vi "Configure Rx Parameters.vi"(6 "rx_gains":dbl[](array[numeric]), 7 "rx_freqs":dbl[](array[numeric]), 8 "error in (no error)":errorcluster, 9 "python path":path, 10 "session in":refnum<k38>, 11 "Refnum in":refnum<k35>) -> (0 "error out":errorcluster, 1 "rx_freqs out":dbl[](array[numeric]), 2 "session out":refnum<k38>, 3 "Refnum out":refnum<k35>)   [LabVIEW 2023]
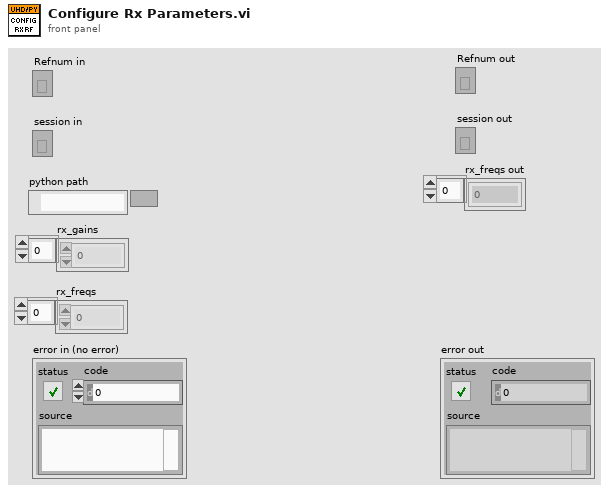
[diagram p1: front panel]
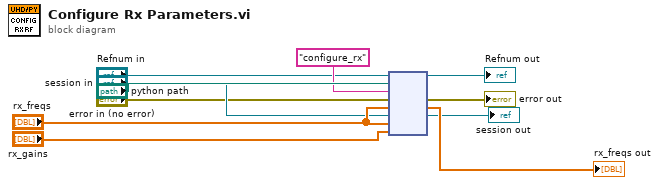
[diagram p0: block diagram]
diagram:
  n1 = node("Refnum in", "python path", "configure_rx" ("function name"), "error in (no error)", "rx_freqs", "session in", "rx_freqs", "rx_gains") -> (→"Refnum out":refnum<k35>, →"error out":errorcluster, →"rx_freqs out":dbl[], →"session out":refnum<k38>)  [unwired: 2 in, 2 out]
